vi "DBC Demo.vi"() -> ()   [LabVIEW 2024]
panel:
  in  "ID":i32=1600 format="%.0x"
  out "signal data":dbl[](array[numeric])=[1.0, -0.87, 0.0, 0.0, 0.27, 0.0, 0.0, 0.0, 0.0, -101.0, 14.200000000000001, 0.0, 27.32, -74.0, 0.0, 1.0, 0.25, 0.0, 0.0, 0.03, 0.0, 0.0, 0.0, 0.0, -101.0, 15.56, 0.0, 19.63, -82.0, 0.0, 0.0, 1.09, 0.0, 0.0, -0.12, 0.0, 0.0, 0.0, 0.0, -101.0, 16.43, 0.0, 18.71, -82.0, 0.0, 0.0, 0.0, 0.0, 0.0, 0.0, 0.0, 0.0, 0.0, 0.0, -255.0, 0.0, 0.0, 0.0, -255.0, 0.0] format="%.2f"
  out "signals":string[](array[string])=["LGU1_azAmb", "LGU1_azAngle", "LGU1_azAngleQly", "LGU1_elAmb", "LGU1_elAngle", "LGU1_elAngleQly", "LGU1_existProb", "LGU1_locPeerIdx", "LGU1_measStatus", "LGU1_noi", "LGU1_radDist", "LGU1_radVel", "LGU1_rcsEst", "LGU1_sigPwr", "LGU1_velQly", "LGU2_azAmb", "LGU2_azAngle", "LGU2_azAngleQly", "LGU2_elAmb", "LGU2_elAngle", "LGU2_elAngleQly", "LGU2_existProb", "LGU2_locPeerIdx", "LGU2_measStatus", "LGU2_noi", "LGU2_radDist", "LGU2_radVel", "LGU2_rcsEst", "LGU2_sigPwr", "LGU2_velQly", "LGU3_azAmb", "LGU3_azAngle", "LGU3_azAngleQly", "LGU3_elAmb", "LGU3_elAngle", "LGU3_elAngleQly", "LGU3_existProb", "LGU3_locPeerIdx", "LGU3_measStatus", "LGU3_noi", "LGU3_radDist", "LGU3_radVel", "LGU3_rcsEst", "LGU3_sigPwr", "LGU3_velQly", "LGU4_azAmb", "LGU4_azAngle", "LGU4_azAngleQly", "LGU4_elAmb", "LGU4_elAngle", "LGU4_elAngleQly", "LGU4_existProb", "LGU4_locPeerIdx", "LGU4_measStatus", "LGU4_noi", "LGU4_radDist", "LGU4_radVel", "LGU4_rcsEst", "LGU4_sigPwr", "LGU4_velQly"]
  in  "payload":u8[](array[numeric])=[140, 5, 0, 0, 0, 205, 218, 172, 202, 134, 212, 0, 0, 0, 0, 0, 20, 6, 0, 0, 0, 205, 214, 171, 199, 128, 12, 0, 0, 0, 0, 0, 107, 6, 0, 0, 0, 205, 86, 79, 7, 253, 54, 0, 0, 0, 0, 0, 0, 0, 0, 0, 0, 0, 0, 0, 0, 0, 0, 0, 0, 0, 0, 0] format="%.0x"
  out "error out":errorcluster
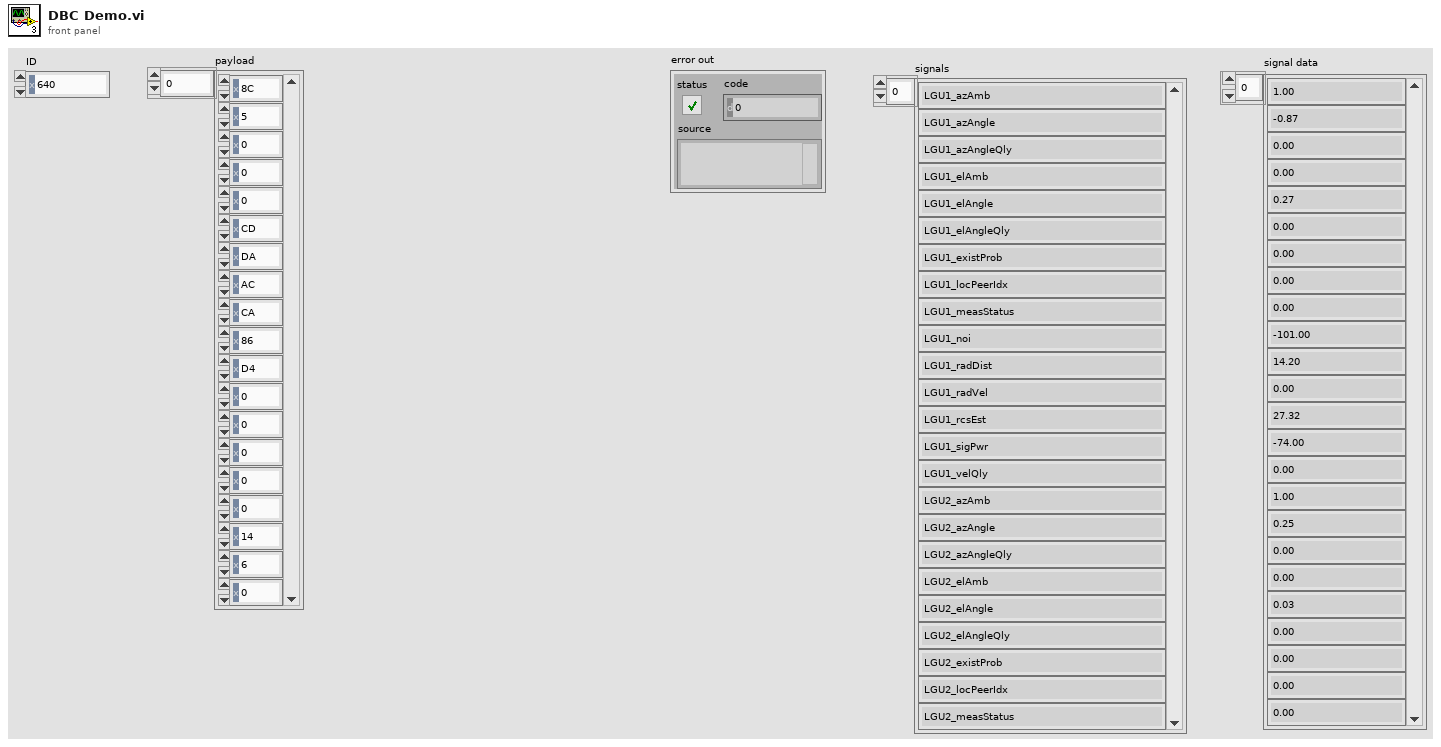
[diagram p1: front panel]
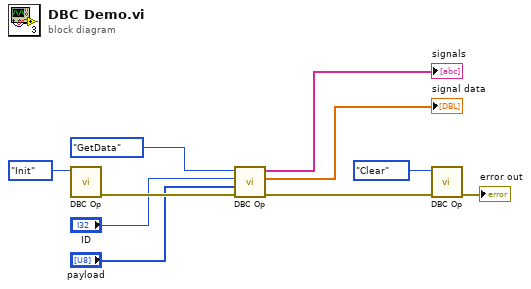
[diagram p0: block diagram]
diagram:
  n1 = call "DBC Op.vi"("Enum"=enum16{"Init", "GetData", "Clear"}."Init") -> ("error out"=w9:errorcluster)  [unwired: 8 in, 2 out]
  n2 = call "DBC Op.vi"("error in (no error)"=w9, "payload"="payload", "ID"="ID", "Enum"=enum16{"Init", "GetData", "Clear"}."GetData") -> ("error out"=w8:errorcluster, "signal data"=→"signal data":dbl[], "signals"=→"signals":string[])  [unwired: 5 in]
  n3 = call "DBC Op.vi"("error in (no error)"=w8, "Enum"=enum16{"Init", "GetData", "Clear"}."Clear") -> ("error out"=→"error out":errorcluster)  [unwired: 7 in, 2 out]
